vi "read Raw.vi"(11 "Path":path) -> (1 "Session Info":T1={"V set"=-1.0, "I compliance"=0.001, "J set"=0.01, "I set"=0.0, "V compliance"=1.0, "Laser Power (mW)"=0.0, "TestID"=0, "Operator"="Radek"} {"V compliance" format="%#_6f"; "I compliance" format="%#_6e"}, 2 "Die Info":T2={"Device Name"="", "ActiveArea_um2"=3848.451, "MesaArea_um2"=3848.451}, 3 "Wafer Info":T3, 4 "V":dbl[](array[numeric]), 6 "I":dbl[](array[numeric]))   [LabVIEW 2012]
uses:
  <vilib>/Utility/file.llb/Read From Spreadsheet File (string).vi
panel:
  in  "Session Info 2":T1={"V set"=-1.0, "I compliance"=0.001, "J set"=0.01, "I set"=0.0, "V compliance"=1.0, "Laser Power (mW)"=0.0, "TestID"=0, "Operator"="Radek"} {"V compliance" format="%#_6f"; "I compliance" format="%#_6e"}
  in  "Die Info 2":T2={"Device Name"="", "ActiveArea_um2"=3848.451, "MesaArea_um2"=3848.451}
  in  "Wafer Info 2":T3
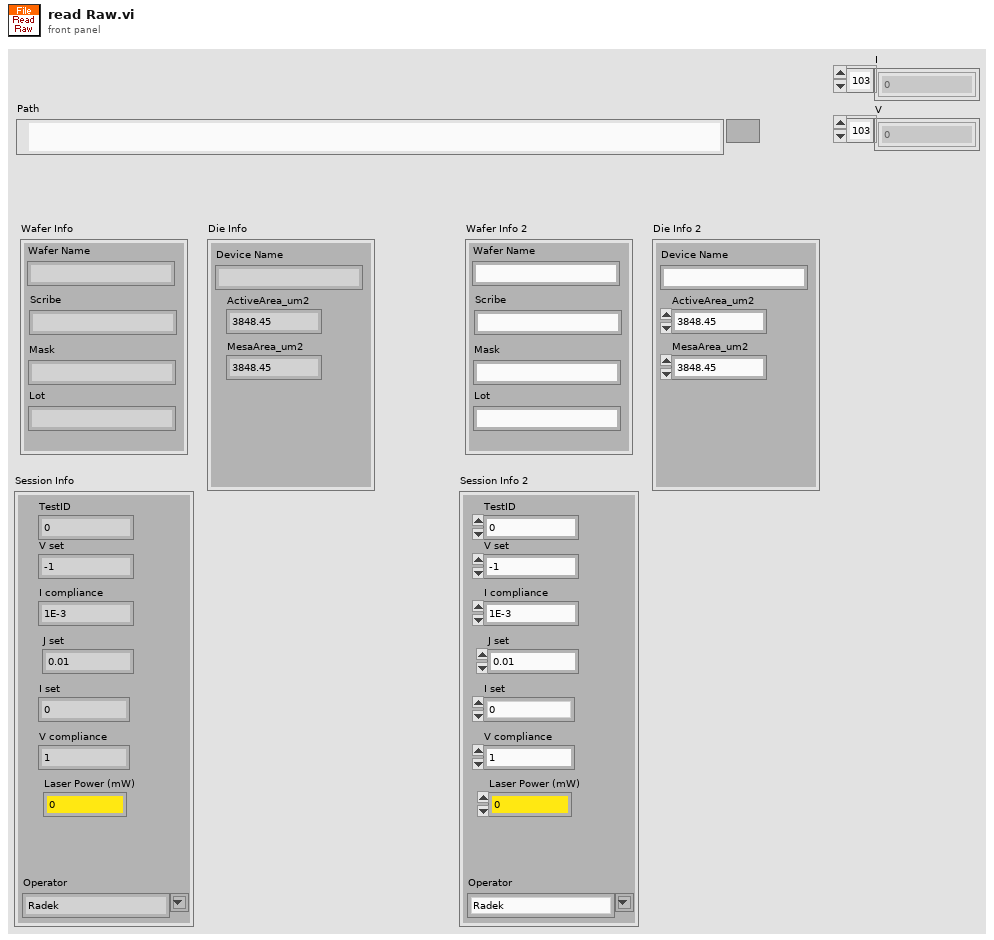
[diagram p1: front panel]
types:
  T1 = cluster{"V set":dbl, "I compliance":dbl, "J set":dbl, "I set":dbl, "V compliance":dbl, "Laser Power (mW)":dbl, "TestID":u32, "Operator":string}
  T2 = cluster{"Device Name":string, "ActiveArea_um2":dbl, "MesaArea_um2":dbl}
  T3 = cluster{"Wafer Name":string, "Scribe":string, "Mask":string, "Lot":string}
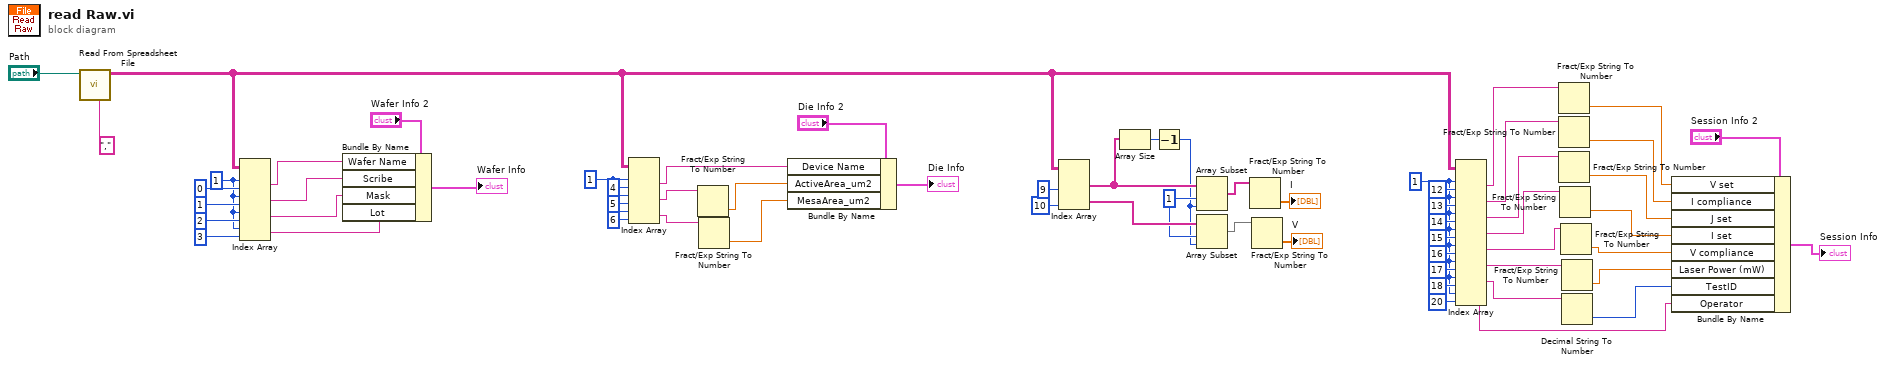
[diagram p0: block diagram]
diagram:
  w10 = 1 ("index (row)")
  w32 = 1 ("index")
  w47 = 1 ("index (row)")
  w52 = 1 ("index")
  n1 = call-poly <vilib>:"Read From Spreadsheet File.vi"("delimiter (\\t)"="," ("delimiter (\\t)"), "file path (dialog if empty)"="Path") -> ("all rows"=w25:string[][])  [unwired: 5 in, 4 out]
  n2 = Index Array(array=w25, index (row) #1=w52, index (col) #1=0 ("disabled index (col)"), index (row) #2=w52, index (col) #2=1 ("disabled index (col)"), index (row) #3=w52, index (col) #3=2 ("disabled index (col)"), index (row) #4=w52, index (col) #4=3 ("disabled index (col)")) -> (element #1=w56:string, element #2=w50:string, element #3=w49:string, element #4=w48:string)
  n3 = Bundle By Name(cluster="Wafer Info 2", "Wafer Name"=w56, "Scribe"=w50, "Mask"=w49, "Lot"=w48) -> (→"Wafer Info":T3)
  n4 = Index Array(array=w25, index (row) #1=w47, index (col) #1=4 ("disabled index (col)"), index (row) #2=w47, index (col) #2=5 ("disabled index (col)"), index (row) #3=w47, index (col) #3=6 ("disabled index (col)")) -> (element #1=w43:string, element #2=w42:string, element #3=w40:string)
  n5 = Fract/Exp String To Number(string=w42) -> (number=w41:dbl)  [unwired: 3 in, 1 out]
  n6 = Fract/Exp String To Number(string=w40) -> (number=w39:dbl)  [unwired: 3 in, 1 out]
  n7 = Bundle By Name(cluster="Die Info 2", "Device Name"=w43, "ActiveArea_um2"=w41, "MesaArea_um2"=w39) -> (→"Die Info":T2)
  n8 = Index Array(array=w25, index (col) #1=9 ("disabled index (col)"), index (col) #2=10 ("index (col)")) -> (element #1=w35:string[], element #2=w33:string[])  [unwired: 2 in]
  n9 = Array Size(array=w35) -> (size(s)=w34:i32)
  n10 = Decrement(x=w34) -> (x-1=w31:i32)
  n11 = Array Subset(array=w35, index=w32, length=w31) -> (w30:string[])
  n12 = Array Subset(array=w33, index=w32, length=w31) -> (w29:string[])
  n13 = Fract/Exp String To Number(string=w30) -> (number=→"I":dbl[])  [unwired: 3 in, 1 out]
  n14 = Fract/Exp String To Number(string=w29) -> (number=→"V":dbl[])  [unwired: 3 in, 1 out]
  n15 = Index Array(array=w25, index (row) #1=w10, index (col) #1=12 ("disabled index (col)"), index (row) #2=w10, index (col) #2=13 ("disabled index (col)"), index (row) #3=w10, index (col) #3=14 ("disabled index (col)"), index (row) #4=w10, index (col) #4=15 ("disabled index (col)"), index (row) #5=w10, index (col) #5=16 ("disabled index (col)"), index (row) #6=w10, index (col) #6=17 ("disabled index (col)"), index (row) #7=w10, index (col) #7=18 ("disabled index (col)"), index (row) #8=w10, index (col) #8=20 ("disabled index (col)")) -> (element #1=w23:string, element #2=w20:string, element #3=w18:string, element #4=w9:string, element #5=w8:string, element #6=w7:string, element #7=w3:string, element #8=w1:string)
  n16 = Fract/Exp String To Number(string=w23) -> (number=w22:dbl)  [unwired: 3 in, 1 out]
  n17 = Fract/Exp String To Number(string=w20) -> (number=w19:dbl)  [unwired: 3 in, 1 out]
  n18 = Fract/Exp String To Number(string=w18) -> (number=w16:dbl)  [unwired: 3 in, 1 out]
  n19 = Fract/Exp String To Number(string=w9) -> (number=w6:dbl)  [unwired: 3 in, 1 out]
  n20 = Fract/Exp String To Number(string=w8) -> (number=w5:dbl)  [unwired: 3 in, 1 out]
  n21 = Fract/Exp String To Number(string=w7) -> (number=w4:dbl)  [unwired: 3 in, 1 out]
  n22 = Decimal String To Number(string=w3) -> (number=w2:i32)  [unwired: 2 in, 1 out]
  n23 = Bundle By Name(cluster="Session Info 2", "V set"=w22, "I compliance"=w19, "J set"=w16, "I set"=w6, "V compliance"=w5, "Laser Power (mW)"=w4, "TestID"=w2, "Operator"=w1) -> (→"Session Info":T1)
